vi "Fiducial Match.vi"(8 "error in (no error)":errorcluster, 10 "input cluster":T1, 11 "Gantry In":refnum<k24>) -> (0 "error out":errorcluster, 1 "Not Found?":bool, 2 "output cluster":T1, 3 "Gantry Out":refnum<k24>)   [LabVIEW 2021, in "Component Tray.lvclass"]
uses:
  Component Tray.lvclass
  Find Component.ctl
  Controller/Camera/Machine Vision.ctl
  C:/Program Files (x86)/Aerotech/A3200/LabVIEW/2010/Bin/Aerotech.A3200.dll
  Program Files (x86)/Aerotech/A3200/LabVIEW/2010/Bin/Aerotech.A3200.dll
  Controller/Motion/A3200/A3200.lvclass
  Controller/Camera/Camera.lvclass
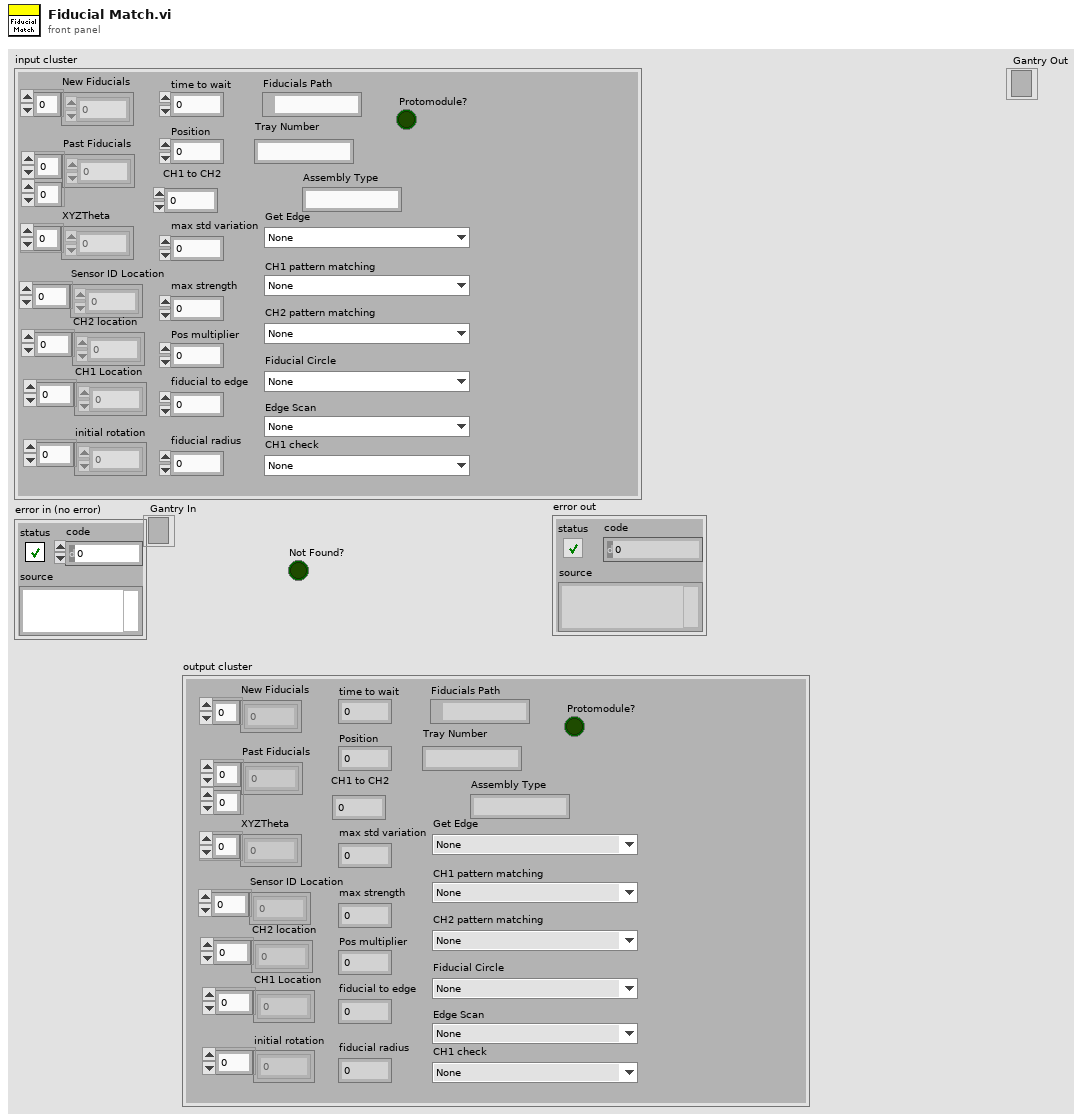
[diagram p1: front panel]
types:
  T1 = typedef "Component Tray.lvclass/Find Component.ctl" = cluster{"New Fiducials":dbl[], "Past Fiducials":dbl[][], "XYZTheta":dbl[], "Fiducials Path":path, "Position":i32, "CH1 Location":dbl[], "Sensor ID Location":dbl[], "initial rotation":dbl[], "CH2 location":dbl[], "max std variation":dbl, "max strength":dbl, "CH2 pattern matching":T2, "Fiducial Circle":T2, "Get Edge":T2, "Pos multiplier":dbl, "time to wait":u32, "fiducial to edge":dbl, "Protomodule?":bool, "Assembly Type":string, "CH1 to CH2":dbl, "Tray Number":string, "fiducial radius":dbl, "4 fiducials?":bool, "CH1 check":T2, "Edge Scan":T2, "CH1 pattern matching":T2, "Sensor Thickness":dbl}
  T2 = typedef "Camera.lvclass/Machine Vision.ctl" = enum16{"None", "Assembly Tray Circle", "Assembly Tray Fiducial", "Partial Hexaboard", "sensor edge init", "HB edge init", "sensor edge pos1", "sensor edge pos2", "HB edge pos1", "HB edge pos2", "Sensor CH1-2", "HB CH1", "HB CH2", "V3 Sensor Circle", "Hexaboard Circle", "sensor CH1 check", "HB CH1 check "}
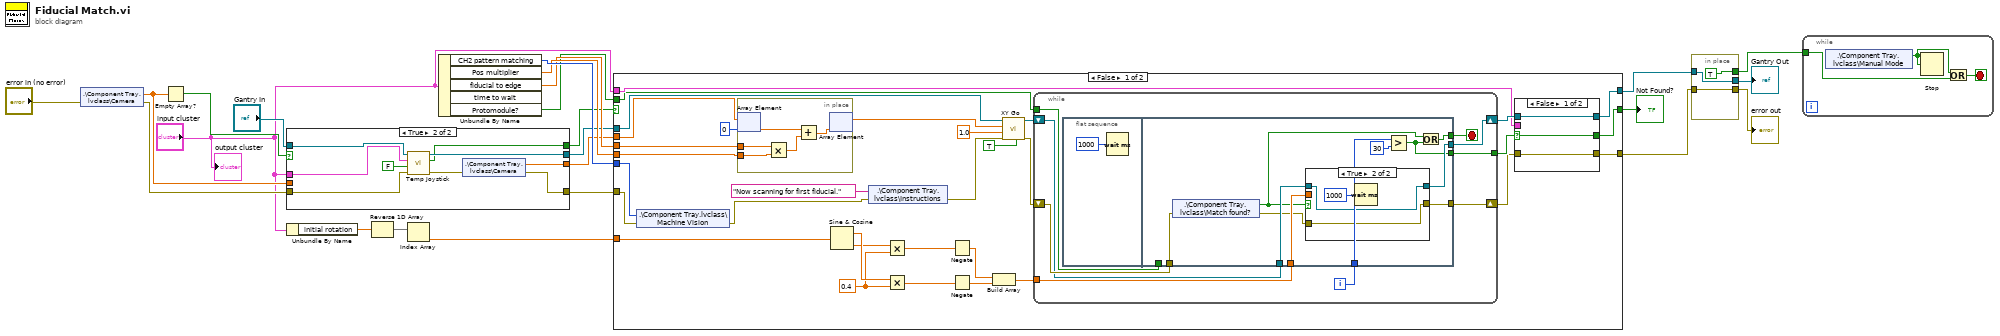
[diagram p0: block diagram]
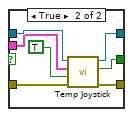
[diagram p2: hidden frame]
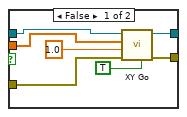
[diagram p3: hidden frame]
diagram:
  n1 = shared-variable ".\\Component Tray.lvclass\\Camera"(error in="error in (no error)") -> (w13:dbl[], error out=w9:errorcluster)
  n2 = Empty Array?(array=w13) -> (empty?=w14:bool)
  n3 = case shown="True" w14 {
    selector: w14 -> [w24 _]
    tunnel: [w27 w29] -> w15
    tunnel: w13 -> [w27 _]
    tunnel: "Gantry In" -> [w26 w36]
    tunnel: [w26 w35] -> w10
    tunnel: "input cluster" -> [_ w34]
    tunnel: w9 -> [w25 w32]
    tunnel: [w25 w30] -> w8
    tunnel: [w24 w28] -> w7
    frame False {
    }
    frame True {
      n4 = call "Temp Joystick.vi"("error in (no error)"=w32, "Fiducial?"=FALSE, "Component"=w34, "Gantry In"=w36) -> ("error out"=w31:errorcluster, "Error?"=w28:bool, "Gantry Out"=w35:refnum<k24>)  [unwired: 5 in]
      n5 = shared-variable ".\\Component Tray.lvclass\\Camera"(error in=w31) -> (w29:dbl[], error out=w30:errorcluster)
    }
  }
  n6 = Unbundle By Name("input cluster") -> ("initial rotation"=w18:dbl[])
  n7 = Reverse 1D Array(array=w18) -> (reversed array=w19:dbl[])
  n8 = Index Array(array=w19) -> (element=w20:dbl)  [unwired: 1 in]
  n9 = Unbundle By Name("input cluster") -> ("CH2 pattern matching"=w23:T2, "Pos multiplier"=w22:dbl, "fiducial to edge"=w21:dbl, "Protomodule?"=w12:bool)  [unwired: 1 out]
  n10 = case shown="False" w7 {
    selector: w7 -> [_ w117]
    tunnel: w23 -> [w68 _]
    tunnel: w22 -> [w65 _]
    tunnel: w21 -> [w64 _]
    tunnel: w20 -> [w61 _]
    tunnel: [w42 w116] -> w4
    tunnel: [w41 w117] -> w17
    tunnel: w15 -> [w56 _]
    tunnel: w12 -> [w38 _]
    tunnel: [w37 w115] -> w1
    tunnel: w10 -> [w46 w116]
    tunnel: w8 -> [w45 w115]
    tunnel: "input cluster" -> [w39 _]
    frame False {
      w58 = 0.4 ("y")
      n11 = shared-variable ".\\Component Tray.lvclass\\Machine Vision"(w68, error in=w45) -> (error out=w47:errorcluster)
      n12 = in-place {
        in-place-border: w65 -> [w112]
        in-place-border: w64 -> [w111]
        n13 = in-place-array #1(w56, 0) -> (w114:dbl)
        n14 = Multiply(x=w111, y=w112) -> (x*y=w113:dbl)
        n15 = Add(x=w114, y=w113) -> (x+y=w110:dbl)
        n16 = in-place-array #1(w110) -> (w63:dbl[])  [unwired: 1 out]
      }
      n17 = Sine & Cosine(0:w61) -> (1:w60:dbl, 2:w59:dbl)
      n18 = shared-variable ".\\Component Tray.lvclass\\Instructions"("Now scanning for first fiducial." ("Instructions"), error in=w47) -> (error out=w48:errorcluster)
      n19 = Multiply(x=w59, y=w58) -> (x*y=w53:dbl)
      n20 = Multiply(x=w60, y=w58) -> (x*y=w55:dbl)
      n21 = Negate(x=w53) -> (-x=w52:dbl)
      n22 = Negate(x=w55) -> (-x=w54:dbl)
      n23 = Build Array(w52, w54) -> (w57:dbl[])
      n24 = call "XY Go.vi"("Increment?"=TRUE, "error in (no error)"=w48, "Speed"=1.0, "XY In"=w63, "Gantry In"=w46) -> ("error out"=w50:errorcluster, "Gantry Out"=w51:refnum<k24>)  [unwired: 4 in, 1 out]
      n25 = while {
        shift-right: [w83] -> w43
        shift-left: w51 -> [w86]
        shift-right: [w84] -> w40
        shift-left: w50 -> [w87]
        tunnel: w57 -> [w85]
        tunnel: [w82] -> w44
        tunnel: w38 -> [w80]
        i -> [w79]
        stop <- w81 stop-if-true
        n26 = flat-sequence {
          tunnel: w87 -> [w95]
          tunnel: w86 -> [w99]
          tunnel: w85 -> [w98]
          tunnel: [w97] -> w84
          tunnel: [w96] -> w83
          tunnel: [w90] -> w82
          tunnel: [w93] -> w81
          tunnel: w80 -> [_]
          tunnel: w79 -> [w91]
          frame #0 {
            n27 = Wait (ms)(milliseconds to wait=u32 1000) -> ()  [unwired: 1 out]
          }
          frame #1 {
            n28 = shared-variable ".\\Component Tray.lvclass\\Match found?"(error in=w95) -> (w92:bool, error out=w94:errorcluster)
            n29 = case shown="True" w92 {
              tunnel: w94 -> [w105 w108]
              tunnel: w99 -> [w103 w109]
              tunnel: [w102 w108] -> w97
              tunnel: [w101 w109] -> w96
              tunnel: w98 -> [w100 _]
              frame False {
                n30 = call "XY Go.vi"("Increment?"=TRUE, "error in (no error)"=w105, "Speed"=1.0, "XY In"=w100, "Gantry In"=w103) -> ("error out"=w102:errorcluster, "Gantry Out"=w101:refnum<k24>)  [unwired: 4 in, 1 out]
              }
              frame True {
                n31 = Wait (ms)(milliseconds to wait=u32 1000) -> ()  [unwired: 1 out]
              }
            }
            n32 = Greater?(x=w91, y=30) -> (0:w90:bool)
            n33 = Or(x=w92, y=w90) -> (x .or. y?=w93:bool)
          }
        }
      }
      n34 = case shown="False" w44 {
        selector: w44 -> [w69 _]
        tunnel: w43 -> [w71 w78]
        tunnel: [w71 w77] -> w42
        tunnel: [w69 w76] -> w41
        tunnel: w40 -> [w70 w74]
        tunnel: [w70 w73] -> w37
        tunnel: w39 -> [_ w72]
        frame False {
        }
        frame True {
          n35 = call "Temp Joystick.vi"("error in (no error)"=w74, "Fiducial?"=TRUE, "Component"=w72, "Gantry In"=w78) -> ("error out"=w73:errorcluster, "Error?"=w76:bool, "Gantry Out"=w77:refnum<k24>)  [unwired: 5 in]
        }
      }
    }
    frame True {
    }
  }
  "Not Found?" <- w17
  n36 = in-place {
    in-place-border: w1 -> [w120]
    in-place-border: [w120] -> w2
    in-place-border: [TRUE ("y")] -> w5
    in-place-border: [w118] -> w3
    in-place-border: w4 -> [w118]
  }
  "Gantry Out" <- w3
  "error out" <- w2
  n37 = while {
    tunnel: w5 -> [w121]
    stop <- w123 stop-if-true
    n38 = shared-variable ".\\Component Tray.lvclass\\Manual Mode"() -> (w122:bool)  [unwired: 1 in, 1 out]
    n39 = Stop(stop? (T)=w122) -> ()
    n40 = Or(x=w122, y=w121) -> (x .or. y?=w123:bool)
  }
  "output cluster" <- "input cluster"
